vi "SoftFrontPanel.vi"(8 "error in (no error)":errorcluster, 11 "DMM Instrument":refnum<class "DMM Instrument.lvclass">) -> (0 "error out":errorcluster, 3 "DMM Instrument out":refnum<class "DMM Instrument.lvclass">)   [LabVIEW 2025, in "DMM.lvlib" / "DMM Instrument.lvclass"]
doc: "Copyright 2017 National Instruments Corporation\n\nLicensed under the Apache License, Version 2.0 (the \"License\"); you may not use this file except in compliance with the License. You may obtain a copy of the License at http://www.apache.org/licenses/LICENSE-2.0\nUnless required by applicable law or agreed to in writing, software distributed under the License is distributed on an \"AS IS\" BASIS, WITHOUT WARRANTIES OR CONDITIONS OF ANY KIND, either express or implied. See the License for the specific language governing permissions and limitations under the License."
uses:
  DMM Instrument.lvclass
  C:/Users/Public/Documents/Sandia National Labs/TSS Plugin/CEF.lvlibp/Node/CEF_Node.lvclass
  DMM Instrument.lvclass/DMM Instrument.ctl
  <vilib>/Analysis/baseanly.llb/Mean (DBL).vi
  DMM configuration/DMM configuration.lvclass
  C:/Users/Public/Documents/Sandia National Labs/TSS Plugin/Abstract Engine.lvlibp/Instrument configuration/Instrument configuration.lvclass
  Users/Public/Documents/Sandia National Labs/TSS Plugin/Abstract Engine.lvlibp/Instrument configuration/Read Instrument Setting.vi
  Users/Public/Documents/Sandia National Labs/TSS Plugin/CEF.lvlibp/Node/ReadChildren.vi
  Users/Public/Documents/Sandia National Labs/TSS Plugin/CEF.lvlibp/Node/CEF_Node.lvclass
  <vilib>/Analysis/NI_AALBase.lvlib
panel:
  in  "Channels":enum32{"Ch0", "Ch1", "Ch2", "Ch3"}(radio)
  out "Instrument":cluster{"Chname":string, "Voltage":dbl}={"Chname"="Ch0", "Voltage"=0.0} {"Voltage" format="%#_4f"}
  out "Instrument":string caption="Instrument ::"
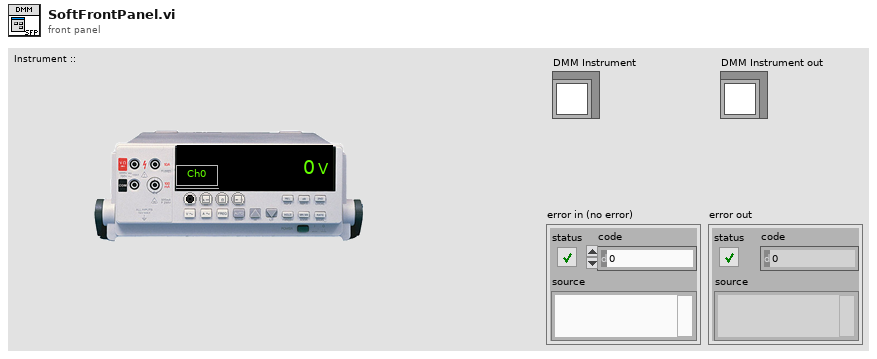
[diagram p1: front panel]
types:
  T1 = enum32{"Invalid", "Default", "Floating", "Floating/Auto-Hide", "Modal"}
  T2 = typedef "Abstract Engine.lvlibp/Instrument configuration.lvclass/Default Instrument.ctl" = cluster{"Type":string, "Address":string, "SW Alias":string, "Description":string, "Enabled":bool}
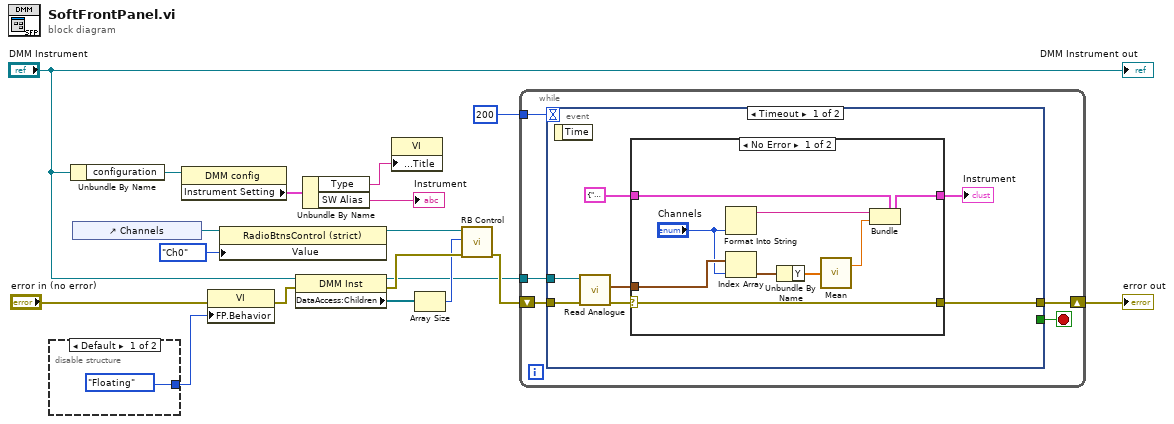
[diagram p0: block diagram]
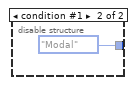
[diagram p2: hidden frame]
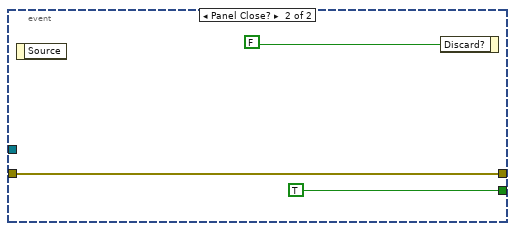
[diagram p4: hidden frame]
diagram:
  n1 = disable-structure shown="Default" {
    disable-tunnel: [T1."Floating" ("Front Panel Window:Behavior") T1."Modal" ("Front Panel Window:Behavior")] -> w16
    frame condition #0 (active) {
    }
    frame condition #1 {
    }
  }
  n2 = Unbundle By Name("DMM Instrument") -> ("configuration"=w14:refnum<class "DMM configuration.lvclass">)
  n3 = control-ref of="Channels"() -> (w6:refnum<vi>)
  n4 = property class="DMM config"(reference=w14) -> ("Instrument Setting"=w13:T2)  [unwired: 1 in, 2 out]
  n5 = property class="VI"(error in="error in (no error)", "FP.Behavior"=w16) -> (error out=w11:errorcluster)  [unwired: 1 in, 1 out]
  n6 = property class="RadioBtnsControl (strict)"(reference=w6, "Value"=enum32{"Ch0", "Ch1", "Ch2", "Ch3"}."Ch0") -> (reference out=w2:refnum<vi>)  [unwired: 1 in, 1 out]
  n7 = property class="DMM Inst"(reference="DMM Instrument", error in=w11) -> (reference out=w4:refnum<class "DMM Instrument.lvclass">, error out=w9:errorcluster, "DataAccess:Children"=w10:refnum<data-value>[])
  n8 = Unbundle By Name(w13) -> ("Type"=w12:string, "SW Alias"=→"Instrument":string)
  n9 = property class="VI"("Front Panel.Title"=w12) -> ()  [unwired: 2 in, 2 out]
  n10 = Array Size(array=w10) -> (size(s)=w7:i32)
  n11 = call "RB Control.vi"("error in"=w9, "Channels"=w7, "Radio Ref"=w2) -> ("error out"=w8:errorcluster)  [unwired: 8 in]
  n12 = while {
    shift-right: [w23] -> w18
    shift-left: w8 -> [w24]
    tunnel: 200 -> [w22]
    tunnel: w4 -> [w21]
    stop <- w25 stop-if-true
    n13 = event shown="[0] Timeout" {
      selector: _ -> [_ _]
      dyn-events: _ -> [_ _]
      timeout: w22 -> [_ _]
      tunnel: [_ TRUE] -> w25
      tunnel: [w26 w43] -> w23
      tunnel: w24 -> [w32 w43]
      tunnel: w21 -> [w31 _]
      event Timeout {
        n14 = event-data() -> ()  [unwired: 1 in, 1 out]
        n15 = call-dynamic "Read Analogue.vi"("error in (no error)"=w32, "Abstract DMM in"=w31) -> ("error out"=w28:errorcluster, "Waveforms"=w29:waveform(dbl)[])  [unwired: 7 in, 1 out]
        n16 = case shown="No Error" w28 {
          selector: w28 -> [w33 _]
          tunnel: [w41 w42] -> w30
          tunnel: w29 -> [w40 _]
          tunnel: cluster{string, "mean":dbl} {"", "mean"=nan} -> [w34 w42]
          tunnel: [w33 _] -> w26
          frame No Error {
            n17 = Format Into String("Channels") -> (resulting string=w39:string)  [unwired: 3 in, 1 out]
            n18 = Index Array(array=w40, index="Channels") -> (element=w37:waveform(dbl))
            n19 = Unbundle By Name(w37) -> ("Y"=w36:dbl[])
            n20 = call-poly <vilib>:"Mean.vi"("X"=w36) -> ("mean"=w35:dbl)  [unwired: 1 out]
            n21 = Bundle(cluster=w34, w39, "mean"=w35) -> (w41:cluster{string, "mean":dbl})
          }
          frame Error {
          }
        }
        "Instrument" <- w30
      }
      event Panel Close? {
        n22 = event-data() -> ()  [unwired: 1 in, 1 out]
        n23 = event-data("Discard?"=FALSE) -> ()  [unwired: 1 in, 1 out]
      }
    }
  }
  "error out" <- w18
  "DMM Instrument out" <- "DMM Instrument"
